vi "depths to intensity.vi"(0 "Display State In":T1={"control refs"={"z offset"=refnum, "laser intensity"=refnum, "XY graph"=refnum}, "error"={"status"=FALSE, "code"=0, "source"=""}, "free-run?"=TRUE, "settings"={"fix points"=[], "A"=0.0, "lambda"=0.0, "C"=0.0}, "range (um)"=400, "interpolate?"=FALSE}, 5 "depth":dbl[unit][](array[numeric]), 9 "Container State":T4, 11 "error in (no error)":errorcluster) -> (4 "Display State Out":T1={"control refs"={"z offset"=refnum, "laser intensity"=refnum, "XY graph"=refnum}, "error"={"status"=FALSE, "code"=0, "source"=""}, "free-run?"=TRUE, "settings"={"fix points"=[], "A"=0.0, "lambda"=0.0, "C"=0.0}, "range (um)"=400, "interpolate?"=FALSE}, 6 "intensity":dbl[](array[numeric]), 15 "error out":errorcluster)   [LabVIEW 2010, in "XIntensityCompensation.xctl"]
uses:
  XIntensityCompensation.xctl
  <vilib>/_xctls/Container State.ctl
  state.ctl
  control_refs.ctl
  settings_cluster.ctl
  <vilib>/_xctls/XControlSupport.lvlib
panel:
  # "Add Controls & Indicators that form the parameters of the method here. Hook them to the connector pane. Do not delete the controls & indicators that are already hooked to the connector pane.\n \nTo setup the parameters  for this method, right click on this item in the Project Tree & select \"Configure Method...\"."
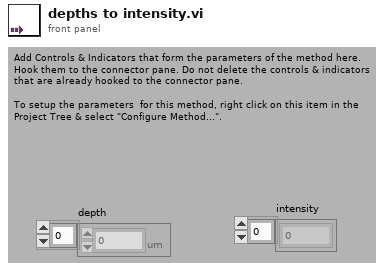
[diagram p1: front panel]
types:
  T1 = typedef "XIntensityCompensation.xctl/state.ctl" = cluster{"control refs":T2, "error":errorcluster, "free-run?":bool, "settings":T3, "range (um)":i32, "interpolate?":bool}
  T2 = typedef "XIntensityCompensation.xctl/control_refs.ctl" = cluster{"z offset":refnum<vi>, "laser intensity":refnum<vi>, "XY graph":refnum<vi>}
  T3 = typedef "XIntensityCompensation.xctl/settings_cluster.ctl" = cluster{"fix points":cluster{"depth":dbl[unit], "intensity":dbl}[], "A":dbl, "lambda":dbl[unit], "C":dbl}
  T4 = typedef "XControlSupport.lvlib/Container State.ctl" = cluster{"Indicator?":bool, "Run Mode?":bool, " Refnum":refnum<vi>}
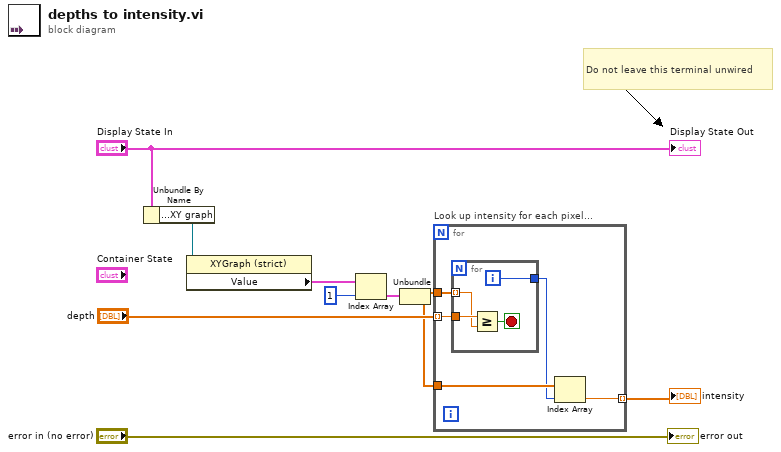
[diagram p0: block diagram]
diagram:
  # "Do not leave this terminal unwired"
  n1 = Unbundle By Name("Display State In") -> ("control refs.XY graph"=w7:refnum<vi>)
  n2 = property class="XYGraph (strict)"(reference=w7) -> ("Value"=w6:cluster{dbl[unit][], dbl[]}[])  [unwired: 1 in, 2 out]
  n3 = Index Array(array=w6, index=1) -> (element=w4:cluster{dbl[unit][], dbl[]})
  n4 = Unbundle(w4) -> (w3:dbl[unit][], w2:dbl[])
  n5 = for "Look up intensity for each pixel..." {
    tunnel: "depth" -> [w15] mode=indexing
    tunnel: w3 -> [w14]
    tunnel: w2 -> [w13]
    tunnel: [w11] -> w1 mode=indexing
    n6 = for {
      tunnel: w15 -> [w19]
      tunnel: w14 -> [w18] mode=indexing
      tunnel: [w16] -> w12
      i -> [w16]
      stop <- w17 stop-if-true
      n7 = Greater Or Equal?(x=w19, y=w18) -> (x >= y?=w17:bool)
    }
    n8 = Index Array(array=w13, index=w12) -> (element=w11:dbl)
  }
  "intensity" <- w1
  "Display State Out" <- "Display State In"
  "error out" <- "error in (no error)"
